vi "Init.vi"(8 "error in (no error)":errorcluster, 11 "Nestle  Actor in":refnum<class "Nestle  Actor.lvclass">) -> (0 "error out":errorcluster, 3 "Nestle  Actor out":refnum<class "Nestle  Actor.lvclass">)   [LabVIEW 2020, in "Nestle  Actor.lvlib" / "Nestle  Actor.lvclass"]
uses:
  Nestle  Actor.lvclass
  Nestle  Actor.lvclass/Nestle  Actor.ctl
  <vilib>/Utility/config.llb/Write Key (String).vi
  <vilib>/Utility/config.llb/NI_LVConfig.lvlib
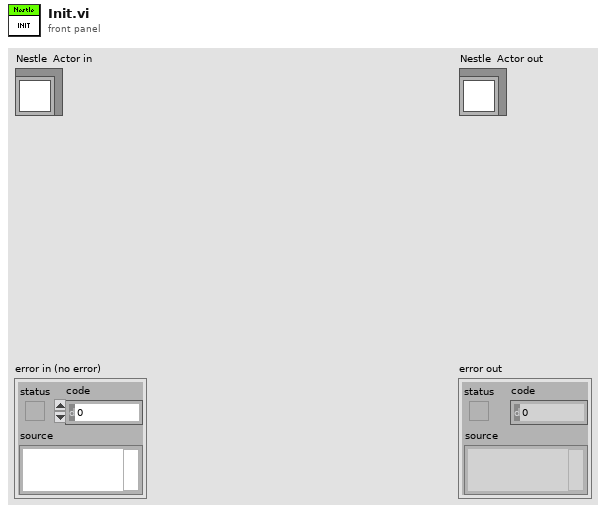
[diagram p1: front panel]
types:
  T1 = typedef "NI_LVConfig.lvlib/Config Data RefNum.ctl" = refnum<k1>
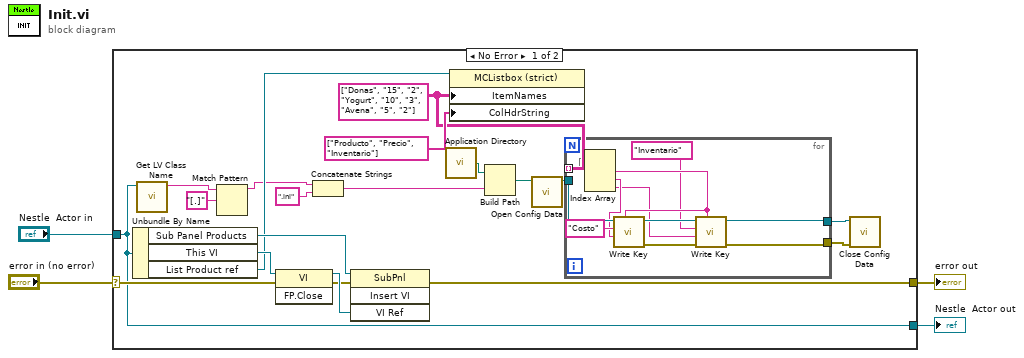
[diagram p0: block diagram]
diagram:
  n1 = case shown="No Error" "error in (no error)" {
    selector: "error in (no error)" -> [w20 w37]
    tunnel: [w19 w37] -> w3
    tunnel: [w16 w36] -> w1
    tunnel: "Nestle  Actor in" -> [w16 w36]
    frame No Error {
      w11 = string[][] [["Donas", "15", "2"], ["Yogurt", "10", "3"], ["Avena", "5", "2"]] ("Item Names")
      n2 = Unbundle By Name(w16) -> ("Sub Panel Products"=w24:refnum<vi>, "This VI"=w23:refnum<vi>, "List Product ref"=w18:refnum<vi>)
      n3 = call <vilib>:"Get LV Class Name.vi"("object"=w16) -> ("class name"=w7:string)  [unwired: 9 in, 1 out]
      n4 = Match Pattern(string=w7, regular expression="[.]") -> (before substring=w6:string)  [unwired: 1 in, 3 out]
      n5 = invoke class="VI" method="FP.Close"(reference=w23, error in=w20) -> (reference out=w22:refnum<vi>, error out=w21:errorcluster)  [unwired: 1 in, 1 out]
      n6 = Concatenate Strings(w6, ".ini" ("string")) -> (w15:string)
      n7 = invoke class="SubPnl" method="Insert VI"(reference=w24, error in=w21, "VI Ref"=w22) -> (error out=w19:errorcluster)  [unwired: 1 in, 3 out]
      n8 = call <vilib>:"Application Directory.vi"() -> ("Application Directory"=w13:path)
      n9 = property class="MCListbox (strict)"(reference=w18, "ItemNames"=w11, "ColHdrString"=string[] ["Producto", "Precio", "Inventario"] ("Column Header Strings[]")) -> ()  [unwired: 1 in, 2 out]
      n10 = Build Path(base path=w13, name or relative path=w15) -> (appended path=w12:path)
      n11 = call <vilib>:"Open Config Data.vi"("configuration file path"=w12) -> ("refnum"=w10:T1)  [unwired: 8 in, 2 out]
      n12 = for {
        tunnel: w11 -> [w30] mode=indexing
        tunnel: w10 -> [w35]
        tunnel: [w32] -> w9
        tunnel: [w31] -> w8
        n13 = Index Array(array=w30) -> (element #1=w29:string, element #2=w26:string, element #3=w25:string)  [unwired: 3 in]
        n14 = call-poly <vilib>:"Write Key.vi"("section"=w29, "value"=w26, "key"="Costo", "refnum"=w35) -> ("error out"=w34:errorcluster, "refnum out"=w33:T1)  [unwired: 5 in, 1 out]
        n15 = call-poly <vilib>:"Write Key.vi"("section"=w29, "error in (no error)"=w34, "value"=w25, "key"="Inventario", "refnum"=w33) -> ("error out"=w31:errorcluster, "refnum out"=w32:T1)  [unwired: 4 in, 1 out]
      }
      n16 = call <vilib>:"Close Config Data.vi"("error in (no error)"=w8, "refnum"=w9) -> ()  [unwired: 8 in, 2 out]
    }
    frame Error {
    }
  }
  "error out" <- w3
  "Nestle  Actor out" <- w1
